vi "Online_TRAC_Add_Measurement.vi"(8 "error in (no error)":errorcluster, 9 "Estimate":dbl format="%#_13g", 10 "True":dbl format="%#_13g", 11 "Online_TRAC in":refnum<class "Online_TRAC.lvclass">) -> (0 "error out":errorcluster, 3 "Online_TRAC out":refnum<class "Online_TRAC.lvclass">)   [LabVIEW 2021, in "Online_TRAC.lvclass"]
uses:
  Online_TRAC.lvclass
  Online_TRAC.lvclass/Online_TRAC.ctl
  Read Square Cross Sum.vi
  Read Square Esitmated Sum.vi
  Read Square True Sum.vi
  Read N.vi
  Write Square Cross Sum.vi
  Write Square Esitmated Sum.vi
  Write Square True Sum.vi
  Write N.vi
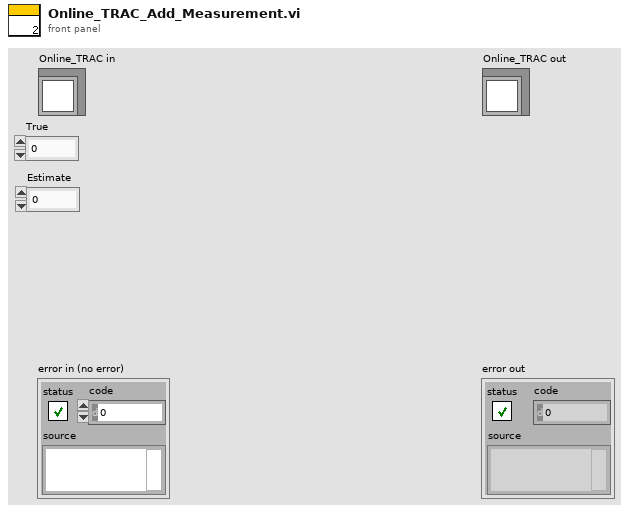
[diagram p1: front panel]
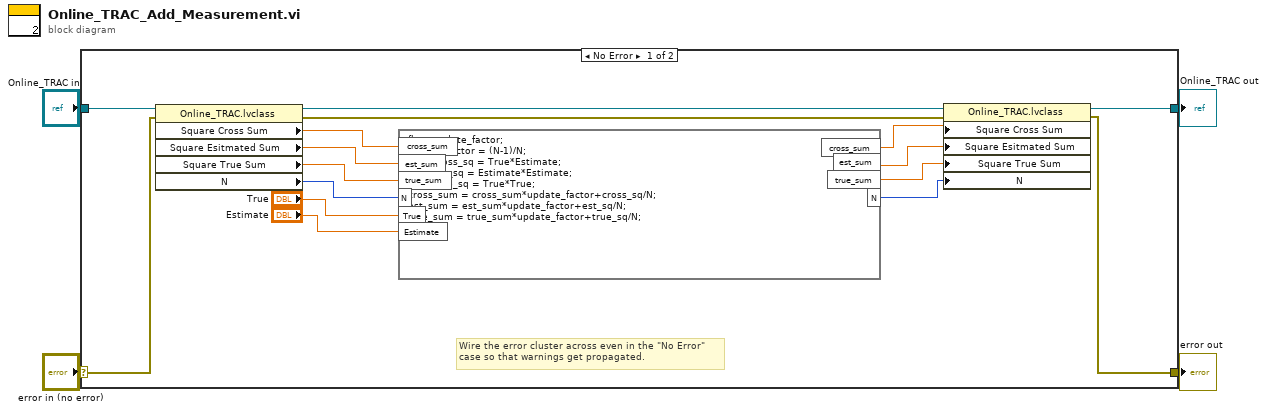
[diagram p0: block diagram]
diagram:
  n1 = case shown="No Error" "error in (no error)" {
    selector: "error in (no error)" -> [w7 w22]
    tunnel: [w8 w21] -> w2
    tunnel: "Online_TRAC in" -> [w9 w21]
    tunnel: [w6 w22] -> w1
    frame No Error {
      # "Wire the error cluster across even in the \"No Error\"\ncase so that warnings get propagated."
      n2 = property class="Online_TRAC.lvclass"(reference=w9, error in=w7) -> (reference out=w11:refnum<class "Online_TRAC.lvclass">, error out=w10:errorcluster, "Square Cross Sum"=w20:dbl, "Square Esitmated Sum"=w19:dbl, "Square True Sum"=w18:dbl, "N"=w17:u64)
      n3 = formula code="float update_factor;\nupdate_factor = (N-1)/N;\nfloat cross_sq = True*Estimate;\nfloat est_sq = Estimate*Estimate;\nfloat true_sq = True*True;\ncross_sum = cross_sum*update_factor+cross_sq/N;\nest_sum = est_sum*update_factor+est_sq/N;\ntrue_sum = true_sum*update_factor+true_sq/N;\nN=N+1;"("cross_sum"=w20, "est_sum"=w19, "true_sum"=w18, "N"=w17, "True"="True", "Estimate"="Estimate") -> ("cross_sum"=w14:dbl, "est_sum"=w13:dbl, "true_sum"=w12:dbl, "N"=w5:u64)
      n4 = property class="Online_TRAC.lvclass"(reference=w11, error in=w10, "Square Cross Sum"=w14, "Square Esitmated Sum"=w13, "Square True Sum"=w12, "N"=w5) -> (reference out=w8:refnum<class "Online_TRAC.lvclass">, error out=w6:errorcluster)
    }
    frame Error {
    }
  }
  "error out" <- w1
  "Online_TRAC out" <- w2
